vi "Path to Images Folder.vi"(8 "Error In":errorcluster) -> (0 "Error Out":errorcluster, 3 "Path To Images Folder":path)   [LabVIEW 2014]
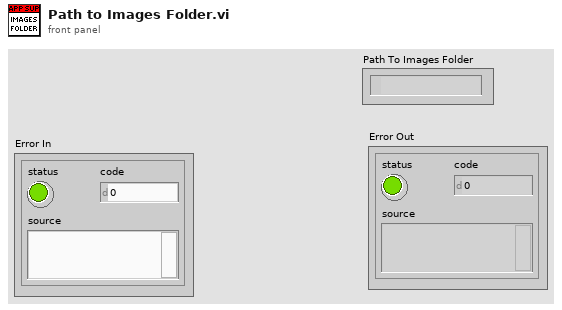
[diagram p1: front panel]
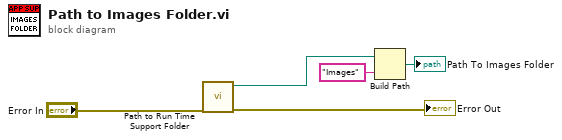
[diagram p0: block diagram]
diagram:
  n1 = call "Path to Run Time Support Folder.vi"("Error In"="Error In") -> ("Error Out"=→"Error Out":errorcluster, "Path To Run Time Support Folder"=w5:path)  [unwired: 9 in]
  n2 = Build Path(base path=w5, name or relative path="Images") -> (appended path=→"Path To Images Folder":path)
